vi "Forward_Kinematics_v2.vi"(1 "theta 3":dbl, 2 "theta 2":dbl, 3 "theta 1":dbl) -> (0 "position":dbl[](array[numeric]))   [LabVIEW 2016]
doc: "This VI takes in the theta 1(deg), theta 2(deg), and theta 3(mm) for L1, L2, and L3 of IRISS. The output will be a position array [px, py, pz]."
uses:
  <vilib>/Analysis/Matrix/Datatypes/RealMatrix.ctl
  <vilib>/Analysis/baseanly.llb/Real A x B.vi
  <vilib>/Analysis/NI_AALBase.lvlib
  <vilib>/Analysis/Matrix/NI_Matrix.lvlib
panel:
  out "T3 mtx":T1
  out "T2 mtx":T1
  out "T1 mtx":T1
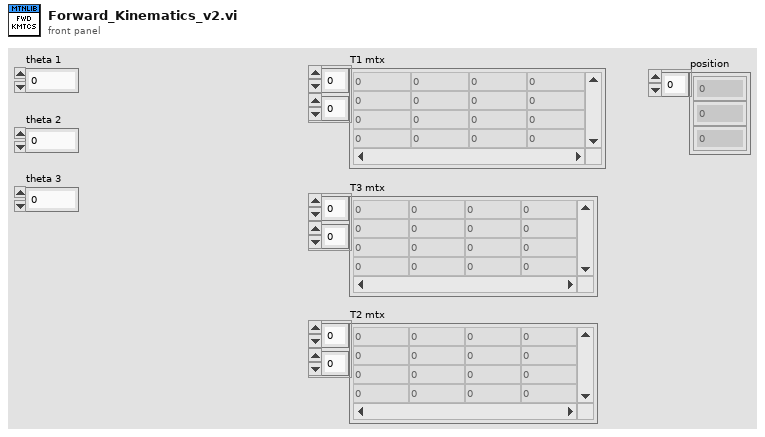
[diagram p1: front panel]
types:
  T1 = typedef "NI_Matrix.lvlib/RealMatrix.ctl" = dbl[][]
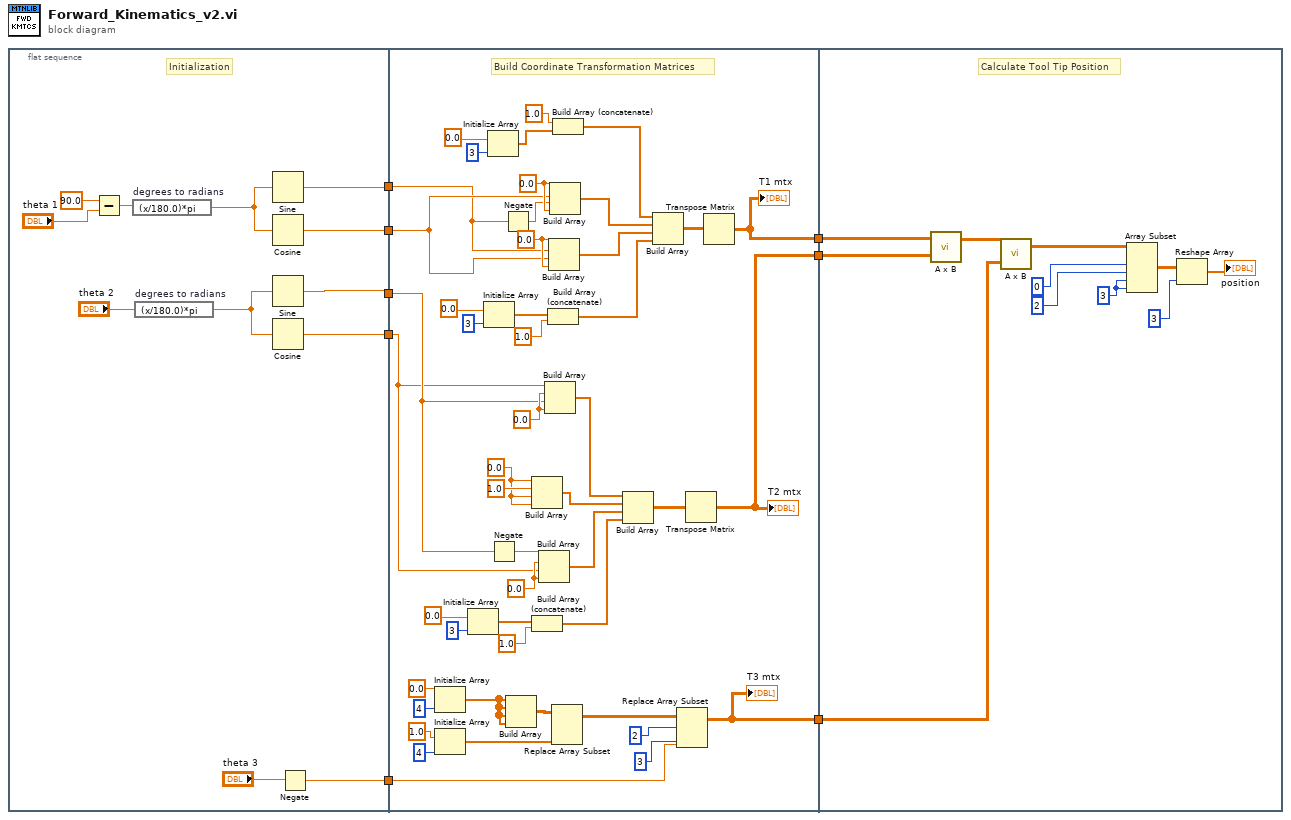
[diagram p0: block diagram]
diagram:
  n1 = flat-sequence {
    tunnel: [w17] -> w8
    tunnel: [w16] -> w7
    tunnel: [w15] -> w6
    tunnel: [w14] -> w5
    tunnel: [w12] -> w4
    tunnel: w8 -> [w28]
    tunnel: w7 -> [w27]
    tunnel: w6 -> [w25]
    tunnel: w5 -> [w26]
    tunnel: w4 -> [w24]
    tunnel: [w23] -> w3
    tunnel: [w22] -> w2
    tunnel: [w21] -> w1
    tunnel: w3 -> [w71]
    tunnel: w2 -> [w70]
    tunnel: w1 -> [w69]
    frame #0 {
      # "Initialization"
      n2 = Subtract(x=90.0, y="theta 1") -> (x-y=w9:dbl)
      n3 = expression code="(x/180.0)*pi" "degrees to radians"(w9) -> (w20:dbl)
      n4 = expression code="(x/180.0)*pi" "degrees to radians"("theta 2") -> (w18:dbl)
      n5 = Sine(x=w20) -> (sin(x)=w16:dbl)
      n6 = Cosine(x=w20) -> (cos(x)=w17:dbl)
      n7 = Sine(x=w18) -> (sin(x)=w14:dbl)
      n8 = Cosine(x=w18) -> (cos(x)=w15:dbl)
      n9 = Negate(x="theta 3") -> (-x=w12:dbl)
    }
    frame #1 {
      w49 = 0.0 ("element")
      w50 = 0.0 ("element")
      w43 = 0.0 ("element")
      w63 = 0.0 ("element")
      w64 = 0.0 ("element")
      # "Build Coordinate Transformation Matrices"
      n10 = Initialize Array(0.0 ("element"), 4 ("dimension size")) -> (w39:dbl[])
      n11 = Initialize Array(1.0 ("element"), 4 ("dimension size")) -> (w35:dbl[])
      n12 = Initialize Array(0.0 ("element"), 3 ("dimension size")) -> (w53:dbl[])
      n13 = Initialize Array(0.0 ("element"), 3 ("dimension size")) -> (w60:dbl[])
      n14 = Initialize Array(0.0 ("element"), 3 ("dimension size")) -> (w67:dbl[])
      n15 = Negate(x=w26) -> (-x=w48:dbl)
      n16 = Negate(x=w27) -> (-x=w31:dbl)
      n17 = Build Array(w39, w39, w39, w39) -> (w38:dbl[][])
      n18 = Build Array(w43, 1.0 ("element"), w43, w43) -> (w46:dbl[])
      n19 = Build Array (concatenate)(w53, 1.0 ("element")) -> (w42:dbl[])
      n20 = Build Array(w48, w49, w25, w49) -> (w45:dbl[])
      n21 = Build Array(w25, w50, w26, w50) -> (w47:dbl[])
      n22 = Build Array (concatenate)(w60, 1.0 ("element")) -> (w55:dbl[])
      n23 = Build Array(w63, w27, w28, w63) -> (w56:dbl[])
      n24 = Build Array(w64, w28, w31, w64) -> (w57:dbl[])
      n25 = Replace Array Subset(array=w38, new element=w35) -> (w34:T1)  [unwired: 2 in]
      n26 = Build Array (concatenate)(1.0 ("element"), w67) -> (w58:dbl[])
      n27 = Build Array(w47, w46, w45, w42) -> (w29:T1)
      n28 = Build Array(w58, w57, w56, w55) -> (w30:T1)
      n29 = Replace Array Subset(array=w34, new element=w24, index (row)=2 ("disabled index (row)"), index (col)=3 ("disabled index (col)")) -> (w21:T1)
      "T3 mtx" <- w21
      n30 = Transpose Matrix(1:w29) -> (0:w22:T1)
      "T2 mtx" <- w22
      n31 = Transpose Matrix(1:w30) -> (0:w23:T1)
      "T1 mtx" <- w23
    }
    frame #2 {
      w75 = 3 ("column 1")
      # "Calculate Tool Tip Position"
      n32 = call-poly <vilib>:"A x B.vi"("B"=w70, "A"=w71) -> ("A x B"=w79:T1)  [unwired: 1 out]
      n33 = call-poly <vilib>:"A x B.vi"("B"=w69, "A"=w79) -> ("A x B"=w78:T1)  [unwired: 1 out]
      n34 = Array Subset(array=w78, index (row)=0 ("row 1"), length (row)=2 ("row N"), index (col)=w75, length (col)=w75) -> (w74:T1)
      n35 = Reshape Array(w74, 3 ("dimension size")) -> (→"position":dbl[])
    }
  }
